vi "2) Programa Control.vi"(0 "VISA resource name":refnum<visa-resource-name>, 1 "error in (no error)":errorcluster) -> (3 "error out":errorcluster)   [LabVIEW 2019]
panel:
  out "Grafica arreglo":string[](array[string])
  in  "Tab Control":enum32{"Page 1"}(tab)
  in  "Refrescar":bool
  out "Gráfica":waveform(dbl)[](graph)
  in  "Guardar imagen":bool
  out "Voltaje":dbl[](array[numeric]) format="%#_4g"
  out "X":dbl[](array[numeric]) format="%#_4g"
  out "Cursores":string[](array[string])
  in  "Título":string
  in  "Guardar txt":bool
  in  "Guardar xls":bool
  in  "Detener":bool
  out "Multiplicadores":dbl[](array[numeric])
  out "Multiplicador":dbl
  out "Multiplicador2":ext
  in  "Acomplamiento":u16(ring) items=["AC", "DC", "GROUND"]
  in  "Atenuación":u16(ring) items=["x1", "x10", "x20", "x50", "x100", "x500", "x1000"]
  in  "Ancho de banda":u16(ring)=1 items=["ON", "OFF"]
  out "Comando 3":string
  in  "Posición vertical":i32(knob) scale=-5.0..5.0
  in  "Escala vertical (V)":u16(ring)=9 items=["2 mV", "5 mV", "10 mV", "20 mV", "50  mV", "100 mV", "200 mV", "500 mV", "1 V", "2 V", "5 V"]
  in  "Invertir canal 2":bool
  in  "Mayor Precisión":bool
  in  "Punto inicial de la onda":i32 min=0 max=2500 step=1
  in  "Punto final de la onda":i32=2500 min=0 max=2500 step=1
  in  "Nivel":ext
  in  "Mode":u16(ring) items=["Auto", "Normal"]
  in  "Estado":bool
  in  "Forzar":bool
  in  "Frecuencia":bool
  out "Comando final Trigger":string
  out "Tipo de trigger":string
  in  "Tipo de Trigger":enum32{"Flanco", "Video", "Pulso"}(tab)
  in  "Canal":u16(ring) items=["Canal 1", "Canal 2"]
  in  "Pendiente":u16(ring)=1 items=["Fall", "Rise"]
  in  "Acoplamiento":u16(ring) items=["AC", "DC", "Sin altas frecuencias DC", "Sin bajas frecuencias AC", "Baja sensibilidad DC"]
  in  "Sync":u16(ring) items=["Field", "Line", "Odd", "Even", "LineNum"]
  in  "Polaridad":u16(ring) items=["Inverted", "Normal"]
  in  "Líneas":dbl(knob) scale=0.0..525.0
  in  "Standard":u16(ring) items=["NTSC", "PAL"]
  in  "Canal":u16(ring) items=["Canal 1", "Canal 2"]
  in  "Width":dbl(knob) scale=3.3e-08..10.0
  in  "When":u16(ring) items=["Equal", "NotEqual", "Inside", "Outside"]
  in  "Polaritdad":u16(ring) items=["Positivo", "Negativo"]
  in  "Ancho":u16(ring) items=["Polarity", "When", "Width"]
  in  "Canal":u16(ring) items=["Canal 1", "Canal 2"]
  in  "Canal MATH":bool
  in  "Canal 1":bool
  in  "Canal 2":bool
  out "Comando 4":string
  out "Comando 2":string
  out "Comando 1":string
  in  "Invertir canal":bool
  in  "Posición horizontal":i32(knob) scale=-5.0..5.0
  in  "Posición vertical":i32(knob) scale=-5.0..5.0
  in  "Escala vertical (V)":u16(ring)=9 items=["2 mV", "5 mV", "10 mV", "20 mV", "50  mV", "100 mV", "200 mV", "500 mV", "1 V", "2 V", "5 V"]
  in  "Escala horizontal (s)":u16(ring)=14 items=["25 n", "50 n", "100 n", "250 n", "500 n", "1 u", "2,5 u", "5 u", "10 u", "25 u", "50 u", "100 u", "250 u", "500 u", "1 m", "2,5 m", "5 m", "10 m", "25 m", "50 m", "100 m", "250 m", "500 m", "1 ", "2,5", "5", "10", "25", "50"]
  in  "Operaciones con las \nseñales (Canal MATH)":u16(ring)=1 items=["CH1 + CH2"=1, "CH1 - CH2"=2, "CH2 - CH1"=3, "CH1 * CH2"=4]
  in  "Acomplamiento":u16(ring) items=["AC", "DC", "GROUND"]
  in  "Atenuación":u16(ring) items=["x1", "x10", "x20", "x50", "x100", "x500", "x1000"]
  in  "Ancho de banda":u16(ring)=1 items=["ON", "OFF"]
  out "Comando concatenado":string
  out "Comando final":string
  # "Opciones avanzadas (trigger)"
  # "Canal 1"
  # "Canal 2"
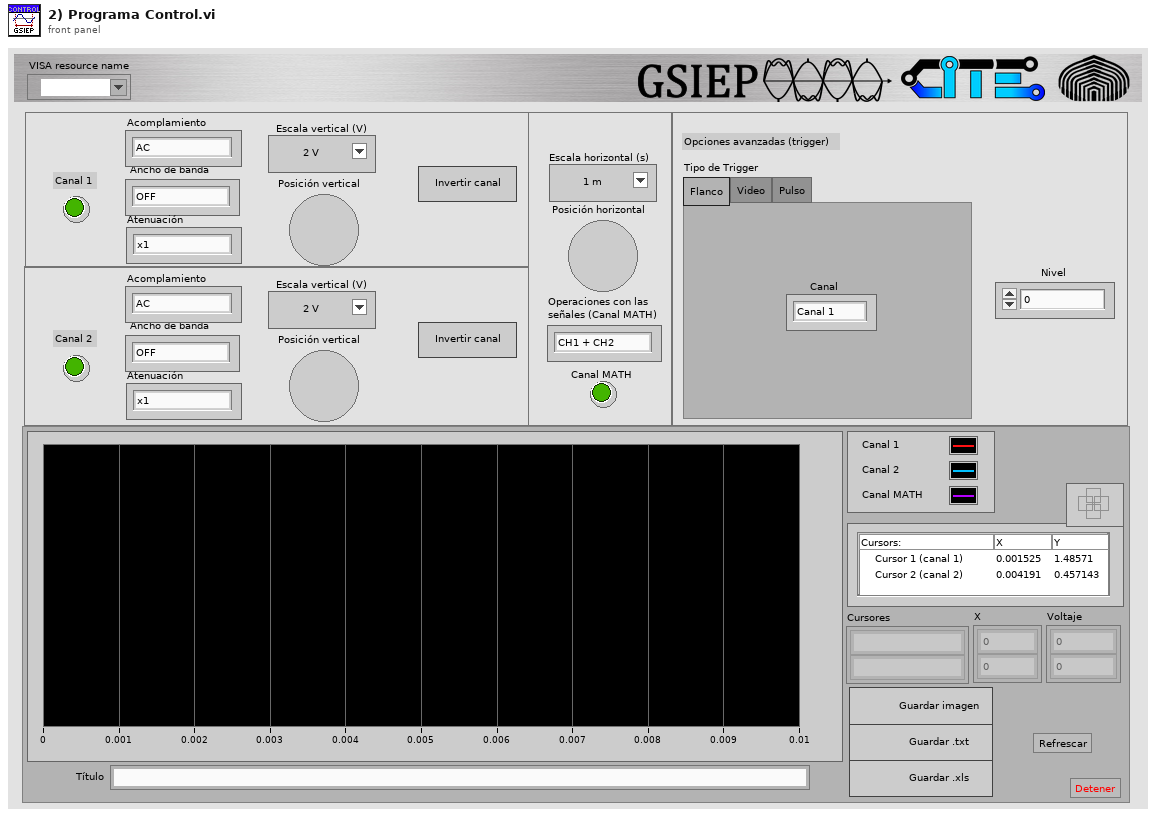
[diagram p1: front panel]
types:
  T1 = cluster{"Canal 1":bool, "Canal 2":bool, "Canal MATH":bool}
  T2 = typedef "LVCursorListTypeDef.ctl" = cluster{"Name":string, "Color":u32, "Style":u8, "Point Style":u8, "Name Visible":bool, "Allow Drag":bool, "Cursor Mode":u32, "Plot":i32, "Index":i32, "Position":cluster{"X":dbl, "Y":dbl}, "X Scale":u32, "Y Scale":u32, "Watch Plots":i32[], "Watch All Plots":bool, "Plot Area":i32, "Label Offset":cluster{"X":dbl, "Y":dbl}}[]
  T3 = typedef "imagedata.ctl" = cluster{"image type":i32, "image depth":i32, "image":u8[], "mask":u8[], "colors":u32[], "Rectangle":cluster{"left":i16, "top":i16, "right":i16, "bottom":i16}}
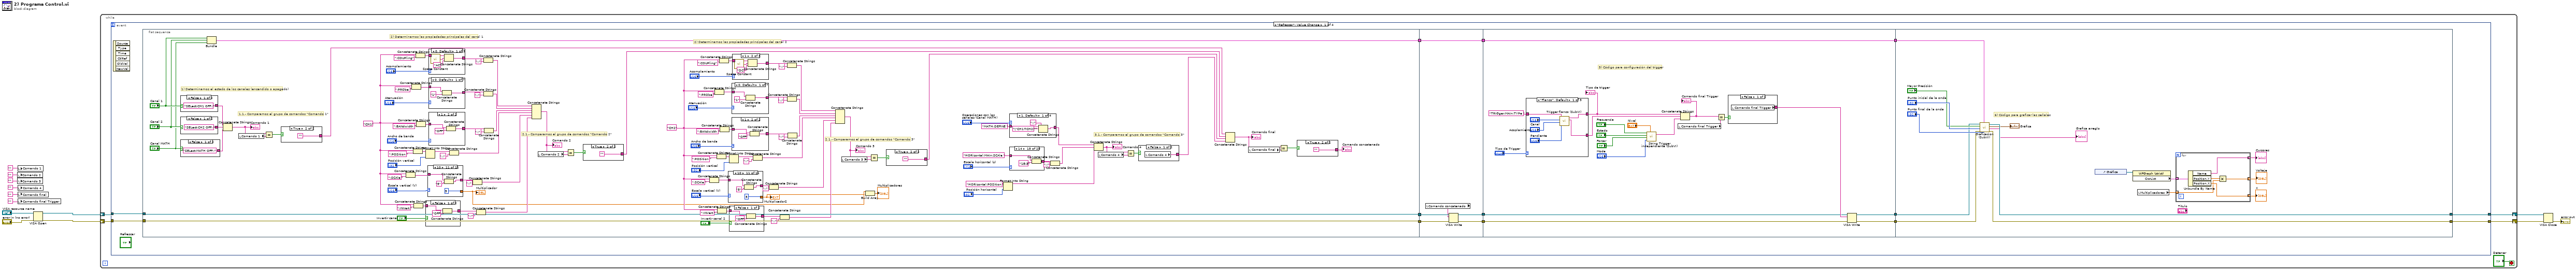
[diagram p0: block diagram]
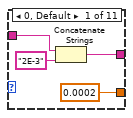
[diagram p2: hidden frame]
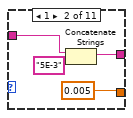
[diagram p3: hidden frame]
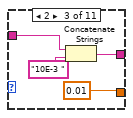
[diagram p4: hidden frame]
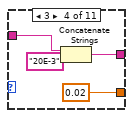
[diagram p5: hidden frame]
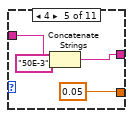
[diagram p6: hidden frame]
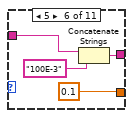
[diagram p7: hidden frame]
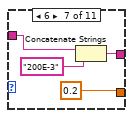
[diagram p8: hidden frame]
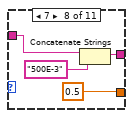
[diagram p9: hidden frame]
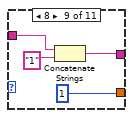
[diagram p10: hidden frame]
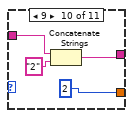
[diagram p11: hidden frame]
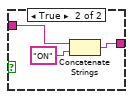
[diagram p12: hidden frame]
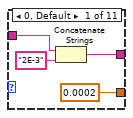
[diagram p13: hidden frame]
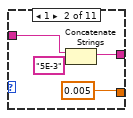
[diagram p14: hidden frame]
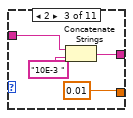
[diagram p15: hidden frame]
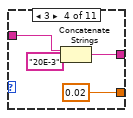
[diagram p16: hidden frame]
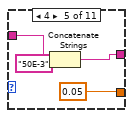
[diagram p17: hidden frame]
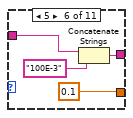
[diagram p18: hidden frame]
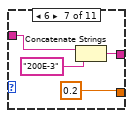
[diagram p19: hidden frame]
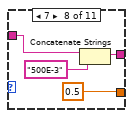
[diagram p20: hidden frame]
diagram:
  n1 = local write "Comando 2"("") -> ()
  n2 = local write "Comando 3"("") -> ()
  n3 = local write "Comando 1"("") -> ()
  n4 = local write "Comando 4"("") -> ()
  n5 = local write "Comando final"("") -> ()
  n6 = local write "Comando final Trigger"("") -> ()
  n7 = VISA Open(error in (no error)="error in (no error)", VISA resource name="VISA resource name") -> (VISA resource name=w2:refnum<visa-resource-name>, error out=w1:errorcluster)  [unwired: 3 in]
  n8 = while {
    shift-right: [w18] -> w13
    shift-left: w2 -> [w16]
    shift-right: [w17] -> w12
    shift-left: w1 -> [w15]
    stop <- "Detener" stop-if-true
    n9 = event shown="[0] \"Refrescar\": Value Change" {
      selector: _ -> [_ _ _ _]
      dyn-events: _ -> [_ _ _ _]
      timeout: _ -> [_ _ _ _]
      tunnel: w16 -> [w22 _ _ _]
      tunnel: w15 -> [w21 _ _ _]
      tunnel: [w20 _ _ _] -> w18
      tunnel: [w19 _ _ _] -> w17
      event "Refrescar": Value Change {
        n10 = event-data() -> ()  [unwired: 1 in, 6 out]
        n11 = flat-sequence {
          tunnel: [w147] -> w30
          tunnel: [w146] -> w29
          tunnel: [w85] -> w31
          tunnel: w22 -> [w147]
          tunnel: w21 -> [w146]
          tunnel: [w448] -> w28
          tunnel: [w447] -> w27
          tunnel: [w446] -> w26
          tunnel: w31 -> [w446]
          tunnel: w30 -> [w445]
          tunnel: w29 -> [w444]
          tunnel: w28 -> [w450]
          tunnel: w27 -> [w449]
          tunnel: w26 -> [w467]
          tunnel: [w453] -> w25
          tunnel: [w452] -> w24
          tunnel: [w467] -> w23
          tunnel: [w501] -> w19
          tunnel: [w502] -> w20
          tunnel: w25 -> [w504]
          tunnel: w24 -> [w503]
          tunnel: w23 -> [w500]
          frame #0 {
            w77 = "CH2"
            w81 = "CH1"
            # "2.1.- Comparamos el grupo de comandos \"Comando 3\""
            # "2) Determinamos las propiedades principales del canal 2"
            # "1) Determinamos el estado de los canales (encendido o apagado)"
            # "3.1.- Comparamos el grupo de comandos \"Comando 3\""
            # "2.1.- Comparamos el grupo de comandos \"Comando 2\""
            # "1.1.- Comparamos el grupo de comandos \"Comando 1\""
            # "2) Determinamos las propiedades principales del canal 1"
            n12 = case shown="False" "Canal 1" {
              tunnel: ["SELect:CH1 OFF;:" "SELect:CH1 ON;:"] -> w143
              frame False {
              }
              frame True {
              }
            }
            n13 = case shown="False" "Canal 2" {
              tunnel: ["SELect:CH2 OFF;:" "SELect:CH2 ON;:"] -> w142
              frame False {
              }
              frame True {
              }
            }
            n14 = case shown="False" "Canal MATH" {
              tunnel: ["SELect:MATH OFF;:" "SELect:MATH ON"] -> w141
              frame False {
              }
              frame True {
              }
            }
            n15 = Bundle("Canal 1"="Canal 1", "Canal 2"="Canal 2", "Canal MATH"="Canal MATH") -> (w85:T1)  [unwired: 1 in]
            n16 = Concatenate Strings(w143, w142, w141) -> (w140:string)
            "Comando 1" <- w140
            n17 = local read "Comando 1"() -> (w139:string)
            n18 = Equal?(x=w140, y=w139) -> (x = y?=w138:bool)
            n19 = case shown="True" w138 {
              tunnel: [w433 ""] -> w94
              frame False {
                n20 = local read "Comando 1"() -> (w433:string)
              }
              frame True {
              }
            }
            n21 = Concatenate Strings(w81, ":SCAle ") -> (w37:string)
            n22 = Concatenate Strings(w81, ":PRObe ") -> (w134:string)
            n23 = Concatenate Strings(w81, ":POSition ") -> (w107:string)
            n24 = Concatenate Strings(w81, ":INVert ") -> (w98:string)
            n25 = Concatenate Strings(w81, ":COUPling") -> (w137:string)
            n26 = Concatenate Strings(w81, ":BANdwidth ") -> (w132:string)
            n27 = Format Into String(initial string=w107, "Posición vertical") -> (resulting string=w112:string)  [unwired: 2 in, 1 out]
            n28 = case shown="False" "Invertir canal" {
              tunnel: w98 -> [w285 w288]
              tunnel: [w284 w287] -> w95
              frame False {
                n29 = Concatenate Strings(w285, "OFF") -> (w284:string)
              }
              frame True {
                n30 = Concatenate Strings(w288, "ON") -> (w287:string)
              }
            }
            n31 = case shown="10" "Escala vertical (V)" {
              tunnel: w37 -> [w151 w156 w159 w163 w167 w171 w174 w179 w183 w187 w191]
              tunnel: [w150 w154 w158 w162 w166 w170 w175 w178 w182 w186 w190] -> w35
              tunnel: [0.0002 0.005 0.01 0.02 0.05 0.1 0.2 0.5 1 2 5] -> w34
              frame 0, Default {
                n32 = Concatenate Strings(w151, "2E-3") -> (w150:string)
              }
              frame 1 {
                n33 = Concatenate Strings(w156, "5E-3") -> (w154:string)
              }
              frame 2 {
                n34 = Concatenate Strings(w159, "10E-3 ") -> (w158:string)
              }
              frame 3 {
                n35 = Concatenate Strings(w163, "20E-3") -> (w162:string)
              }
              frame 4 {
                n36 = Concatenate Strings(w167, "50E-3") -> (w166:string)
              }
              frame 5 {
                n37 = Concatenate Strings(w171, "100E-3") -> (w170:string)
              }
              frame 6 {
                n38 = Concatenate Strings(w174, "200E-3") -> (w175:string)
              }
              frame 7 {
                n39 = Concatenate Strings(w179, "500E-3") -> (w178:string)
              }
              frame 8 {
                n40 = Concatenate Strings(w183, "1") -> (w182:string)
              }
              frame 9 {
                n41 = Concatenate Strings(w187, "2") -> (w186:string)
              }
              frame 10 {
                n42 = Concatenate Strings(w191, "5") -> (w190:string)
              }
            }
            "Multiplicador" <- w34
            n43 = case shown="0, Default" "Atenuación" {
              tunnel: w134 -> [w401 w405 w407 w410 w413 w416 w419]
              tunnel: [w400 w403 w406 w409 w412 w415 w418] -> w123
              frame 0, Default {
                n44 = Concatenate Strings(w401, "1") -> (w400:string)
              }
              frame 1 {
                n45 = Concatenate Strings(w405, "10") -> (w403:string)
              }
              frame 2 {
                n46 = Concatenate Strings(w407, "20") -> (w406:string)
              }
              frame 3 {
                n47 = Concatenate Strings(w410, "50") -> (w409:string)
              }
              frame 4 {
                n48 = Concatenate Strings(w413, "100") -> (w412:string)
              }
              frame 5 {
                n49 = Concatenate Strings(w416, "500") -> (w415:string)
              }
              frame 6 {
                n50 = Concatenate Strings(w419, "1000") -> (w418:string)
              }
            }
            n51 = case shown="1" "Ancho de banda" {
              tunnel: w132 -> [w396 w399]
              tunnel: [w394 w397] -> w121
              frame 0, Default {
                n52 = Concatenate Strings(w396, "ON") -> (w394:string)
              }
              frame 1 {
                n53 = Concatenate Strings(w399, "OFF") -> (w397:string)
              }
            }
            n54 = case shown="0, Default" "Acomplamiento" {
              tunnel: w137 -> [w422 w425 w430]
              tunnel: [w421 w426 w429] -> w126
              frame 0, Default {
                n55 = call <vilib>:"Space Constant.vi"() -> ("String"=w423:string)
                n56 = Concatenate Strings(w422, w423, "AC") -> (w421:string)
              }
              frame 1 {
                n57 = call <vilib>:"Space Constant.vi"() -> ("String"=w427:string)
                n58 = Concatenate Strings(w425, w427, "DC") -> (w426:string)
              }
              frame 2 {
                n59 = call <vilib>:"Space Constant.vi"() -> ("String"=w431:string)
                n60 = Concatenate Strings(w430, w431, "GND") -> (w429:string)
              }
            }
            n61 = Concatenate Strings(w112, ";:") -> (w84:string)
            n62 = Concatenate Strings(w35, ";:") -> (w83:string)
            n63 = Concatenate Strings(w95, ";:") -> (w80:string)
            n64 = Concatenate Strings(w126, ";:") -> (w91:string)
            n65 = Concatenate Strings(w123, ";:") -> (w90:string)
            n66 = Concatenate Strings(w121, ";:") -> (w89:string)
            n67 = Concatenate Strings(w91, w90, w89, w84, w83, w80) -> (w118:string)
            "Comando 2" <- w118
            n68 = local read "Comando 2"() -> (w119:string)
            n69 = Equal?(x=w118, y=w119) -> (x = y?=w120:bool)
            n70 = case shown="True" w120 {
              tunnel: [w379 ""] -> w93
              frame False {
                n71 = local read "Comando 2"() -> (w379:string)
              }
              frame True {
              }
            }
            n72 = Concatenate Strings(w77, ":SCAle ") -> (w61:string)
            n73 = Concatenate Strings(w77, ":PRObe ") -> (w42:string)
            n74 = Concatenate Strings(w77, ":POSition ") -> (w64:string)
            n75 = Concatenate Strings(w77, ":INVert ") -> (w68:string)
            n76 = Concatenate Strings(w77, ":COUPling") -> (w39:string)
            n77 = Concatenate Strings(w77, ":BANdwidth ") -> (w44:string)
            n78 = case shown="10" "Escala vertical (V)" {
              tunnel: w61 -> [w201 w206 w209 w213 w217 w221 w224 w229 w233 w237 w241]
              tunnel: [w200 w204 w208 w212 w216 w220 w225 w228 w232 w236 w240] -> w65
              tunnel: [0.0002 0.005 0.01 0.02 0.05 0.1 0.2 0.5 1 2 5] -> w33
              frame 0, Default {
                n79 = Concatenate Strings(w201, "2E-3") -> (w200:string)
              }
              frame 1 {
                n80 = Concatenate Strings(w206, "5E-3") -> (w204:string)
              }
              frame 2 {
                n81 = Concatenate Strings(w209, "10E-3 ") -> (w208:string)
              }
              frame 3 {
                n82 = Concatenate Strings(w213, "20E-3") -> (w212:string)
              }
              frame 4 {
                n83 = Concatenate Strings(w217, "50E-3") -> (w216:string)
              }
              frame 5 {
                n84 = Concatenate Strings(w221, "100E-3") -> (w220:string)
              }
              frame 6 {
                n85 = Concatenate Strings(w224, "200E-3") -> (w225:string)
              }
              frame 7 {
                n86 = Concatenate Strings(w229, "500E-3") -> (w228:string)
              }
              frame 8 {
                n87 = Concatenate Strings(w233, "1") -> (w232:string)
              }
              frame 9 {
                n88 = Concatenate Strings(w237, "2") -> (w236:string)
              }
              frame 10 {
                n89 = Concatenate Strings(w241, "5") -> (w240:string)
              }
            }
            "Multiplicador2" <- w33
            n90 = Format Into String(initial string=w64, "Posición vertical") -> (resulting string=w59:string)  [unwired: 2 in, 1 out]
            n91 = case shown="False" "Invertir canal 2" {
              tunnel: w68 -> [w194 w197]
              tunnel: [w193 w196] -> w71
              frame False {
                n92 = Concatenate Strings(w194, "OFF") -> (w193:string)
              }
              frame True {
                n93 = Concatenate Strings(w197, "ON") -> (w196:string)
              }
            }
            n94 = case shown="0, Default" "Atenuación" {
              tunnel: w42 -> [w252 w256 w258 w261 w264 w267 w270]
              tunnel: [w251 w254 w257 w260 w263 w266 w269] -> w51
              frame 0, Default {
                n95 = Concatenate Strings(w252, "1") -> (w251:string)
              }
              frame 1 {
                n96 = Concatenate Strings(w256, "10") -> (w254:string)
              }
              frame 2 {
                n97 = Concatenate Strings(w258, "20") -> (w257:string)
              }
              frame 3 {
                n98 = Concatenate Strings(w261, "50") -> (w260:string)
              }
              frame 4 {
                n99 = Concatenate Strings(w264, "100") -> (w263:string)
              }
              frame 5 {
                n100 = Concatenate Strings(w267, "500") -> (w266:string)
              }
              frame 6 {
                n101 = Concatenate Strings(w270, "1000") -> (w269:string)
              }
            }
            n102 = case shown="1" "Ancho de banda" {
              tunnel: w44 -> [w247 w250]
              tunnel: [w245 w248] -> w53
              frame 0, Default {
                n103 = Concatenate Strings(w247, "ON") -> (w245:string)
              }
              frame 1 {
                n104 = Concatenate Strings(w250, "OFF") -> (w248:string)
              }
            }
            n105 = case shown="1" "Acomplamiento" {
              tunnel: w39 -> [w273 w276 w281]
              tunnel: [w272 w277 w280] -> w48
              frame 0, Default {
                n106 = call <vilib>:"Space Constant.vi"() -> ("String"=w274:string)
                n107 = Concatenate Strings(w273, w274, "AC") -> (w272:string)
              }
              frame 1 {
                n108 = call <vilib>:"Space Constant.vi"() -> ("String"=w278:string)
                n109 = Concatenate Strings(w276, w278, "DC") -> (w277:string)
              }
              frame 2 {
                n110 = call <vilib>:"Space Constant.vi"() -> ("String"=w282:string)
                n111 = Concatenate Strings(w281, w282, "GND") -> (w280:string)
              }
            }
            n112 = Concatenate Strings(w59, ";:") -> (w75:string)
            n113 = Concatenate Strings(w65, ";:") -> (w76:string)
            n114 = Concatenate Strings(w71, ";:") -> (w78:string)
            n115 = Concatenate Strings(w48, ";:") -> (w72:string)
            n116 = Concatenate Strings(w51, ";:") -> (w73:string)
            n117 = Concatenate Strings(w53, ";:") -> (w74:string)
            n118 = Concatenate Strings(w72, w73, w74, w75, w76, w78) -> (w56:string)
            "Comando 3" <- w56
            n119 = local read "Comando 3"() -> (w55:string)
            n120 = Build Array(w34, w33) -> (→"Multiplicadores":dbl[])
            n121 = Equal?(x=w56, y=w55) -> (x = y?=w54:bool)
            n122 = case shown="True" w54 {
              tunnel: [w243 ""] -> w38
              frame False {
                n123 = local read "Comando 3"() -> (w243:string)
              }
              frame True {
              }
            }
            n124 = Format Into String(initial string="HORizontal:POSition ", "Posición horizontal") -> (resulting string=w114:string)  [unwired: 2 in, 1 out]
            n125 = case shown="1, Default" "Operaciones con las \nseñales (Canal MATH)" {
              tunnel: "MATH:DEFINE " -> [w384 w387 w389 w392]
              tunnel: [w382 w386 w388 w391] -> w82
              frame 1, Default {
                n126 = Concatenate Strings(w384, "\"CH1+CH2\"", ";:" ("string")) -> (w382:string)
              }
              frame 2 {
                n127 = Concatenate Strings(w387, "\"CH1-CH2\"") -> (w386:string)
              }
              frame 3 {
                n128 = Concatenate Strings(w389, "\"CH2-CH1\"") -> (w388:string)
              }
              frame 4 {
                n129 = Concatenate Strings(w392, "\"CH1*CH2\"") -> (w391:string)
              }
            }
            n130 = case shown="14" "Escala horizontal (s)" {
              tunnel: "HORizontal:MAIn:SCAle " -> [w293 w297 w299 w302 w305 w308 w311 w314 w317 w320 w323 w325 w328 w331 w334 w337 w340 w343 w346 w349 w352 w355 w358 w361 w364 w367 w370 w373 w376]
              tunnel: [w292 w295 w298 w301 w304 w307 w312 w313 w316 w319 w322 w326 w329 w332 w335 w338 w341 w344 w347 w350 w353 w356 w359 w362 w365 w368 w371 w374 w377] -> w105
              frame 0, Default {
                n131 = Concatenate Strings(w293, "25E-9") -> (w292:string)
              }
              frame 1 {
                n132 = Concatenate Strings(w297, "50E-9") -> (w295:string)
              }
              frame 2 {
                n133 = Concatenate Strings(w299, "100E-9") -> (w298:string)
              }
              frame 3 {
                n134 = Concatenate Strings(w302, "250E-9") -> (w301:string)
              }
              frame 4 {
                n135 = Concatenate Strings(w305, "500E-9") -> (w304:string)
              }
              frame 5 {
                n136 = Concatenate Strings(w308, "1E-6") -> (w307:string)
              }
              frame 6 {
                n137 = Concatenate Strings(w311, "2.5E-6") -> (w312:string)
              }
              frame 7 {
                n138 = Concatenate Strings(w314, "5E-6") -> (w313:string)
              }
              frame 8 {
                n139 = Concatenate Strings(w317, "10E-6") -> (w316:string)
              }
              frame 9 {
                n140 = Concatenate Strings(w320, "25E-6") -> (w319:string)
              }
              frame 10 {
                n141 = Concatenate Strings(w323, "50E-6") -> (w322:string)
              }
              frame 11 {
                n142 = Concatenate Strings(w325, "100E-6") -> (w326:string)
              }
              frame 12 {
                n143 = Concatenate Strings(w328, "250E-6") -> (w329:string)
              }
              frame 13 {
                n144 = Concatenate Strings(w331, "500E-6") -> (w332:string)
              }
              frame 14 {
                n145 = Concatenate Strings(w334, "1E-3") -> (w335:string)
              }
              frame 15 {
                n146 = Concatenate Strings(w337, "2.5E-3") -> (w338:string)
              }
              frame 16 {
                n147 = Concatenate Strings(w340, "5E-3") -> (w341:string)
              }
              frame 17 {
                n148 = Concatenate Strings(w343, "10E-3") -> (w344:string)
              }
              frame 18 {
                n149 = Concatenate Strings(w346, "25E-3") -> (w347:string)
              }
              frame 19 {
                n150 = Concatenate Strings(w349, "50E-3") -> (w350:string)
              }
              frame 20 {
                n151 = Concatenate Strings(w352, "100E-3") -> (w353:string)
              }
              frame 21 {
                n152 = Concatenate Strings(w355, "250E-3") -> (w356:string)
              }
              frame 22 {
                n153 = Concatenate Strings(w358, "500E-3") -> (w359:string)
              }
              frame 23 {
                n154 = Concatenate Strings(w361, "1E0") -> (w362:string)
              }
              frame 24 {
                n155 = Concatenate Strings(w364, "2.5E0") -> (w365:string)
              }
              frame 25 {
                n156 = Concatenate Strings(w367, "5E0") -> (w368:string)
              }
              frame 26 {
                n157 = Concatenate Strings(w370, "10E0") -> (w371:string)
              }
              frame 27 {
                n158 = Concatenate Strings(w373, "25E0") -> (w374:string)
              }
              frame 28 {
                n159 = Concatenate Strings(w376, "50E0") -> (w377:string)
              }
            }
            n160 = Concatenate Strings(w105, ";:") -> (w104:string)
            n161 = Concatenate Strings(w82, w104, w114) -> (w100:string)
            "Comando 4" <- w100
            n162 = local read "Comando 4"() -> (w102:string)
            n163 = Equal?(x=w100, y=w102) -> (x = y?=w101:bool)
            n164 = case shown="False" w101 {
              tunnel: [w290 ""] -> w79
              frame False {
                n165 = local read "Comando 4"() -> (w290:string)
              }
              frame True {
              }
            }
            n166 = Concatenate Strings(w94, w93, w38, w79) -> (w92:string)
            "Comando final" <- w92
            n167 = local read "Comando final"() -> (w145:string)
            n168 = Equal?(x=w92, y=w145) -> (x = y?=w148:bool)
            n169 = case shown="True" w148 {
              tunnel: [w441 ""] -> w144
              frame False {
                n170 = local read "Comando final"() -> (w441:string)
              }
              frame True {
              }
            }
            "Comando concatenado" <- w144
          }
          frame #1 {
            n171 = local read "Comando concatenado"() -> (w443:string)
            n172 = VISA Write(VISA resource name=w445, write buffer=w443, error in (no error)=w444) -> (VISA resource name out=w448:refnum<visa-resource-name>, error out=w447:errorcluster)  [unwired: 1 out]
          }
          frame #2 {
            # "5) Código para configuración del trigger"
            n173 = case shown="\"Flanco\", Default" "Tipo de Trigger" {
              tunnel: "TRIGger:MAIn:TYPe " -> [w474 w480 w491]
              tunnel: [w475 w482 w490] -> w455
              tunnel: [w470 w481 w489] -> w456
              frame "Flanco", Default {
                n174 = call "Trigger flanco (SubVI).vi"("Slope"="Pendiente", "Acoplamiento"="Acoplamiento", "Canal"="Canal", "String de Entrada"=w474) -> ("String de Salida"=w470:string, "String de tipo"=w475:string)  [unwired: 6 in]
              }
              frame "Video" {
                n175 = call "Trigger Video (SubVI).vi"("Sync"="Sync", "Lines"="Líneas", "Standard"="Standard", "Polarity"="Polaridad", "Canal"="Canal", "String de Entrada"=w480) -> ("String de Salida"=w481:string, "String de Tipo"=w482:string)  [unwired: 4 in]
              }
              frame "Pulso" {
                n176 = call "Trigger Pulso (SubVI).vi"("Polarity"="Polaritdad", "Width"="Width", "When"="When", "Ancho"="Ancho", "Canal"="Canal", "String de Entrada"=w491) -> ("String de Salida"=w489:string, "String de Tipo"=w490:string)  [unwired: 4 in]
              }
            }
            "Tipo de trigger" <- w455
            n177 = call "String Trigger independiente (SubVI).vi"("Nivel"="Nivel", "Mode"="Mode", "Force"="Forzar", "State"="Estado", "Frecuency"="Frecuencia") -> ("String trigges independiente"=w466:string)  [unwired: 2 in]
            n178 = local read "Comando final Trigger"() -> (w457:string)
            n179 = Concatenate Strings(w455, w456, w466) -> (w454:string)
            "Comando final Trigger" <- w454
            n180 = Equal?(x=w454, y=w457) -> (x = y?=w458:bool)
            n181 = case shown="False" w458 {
              tunnel: [w468 ""] -> w451
              frame False {
                n182 = local read "Comando final Trigger"() -> (w468:string)
              }
              frame True {
              }
            }
            n183 = VISA Write(VISA resource name=w450, write buffer=w451, error in (no error)=w449) -> (VISA resource name out=w453:refnum<visa-resource-name>, error out=w452:errorcluster)  [unwired: 1 out]
          }
          frame #3 {
            # "6) Código para graficar las señales"
            n184 = call "Graficacion (SubVI).vi"("Punto final de la onda"="Punto final de la onda", "Estados de los canales"=w500, "error in (no error)"=w503, "Punto inicial de la onda"="Punto inicial de la onda", "Mayor Precisión"="Mayor Precisión", "VISA Refnum in"=w504) -> ("error out"=w501:errorcluster, "Array"=→"Grafica arreglo":string[], "Gráfica"=→"Gráfica":waveform(dbl)[], "VISA Refnum out"=w502:refnum<visa-resource-name>)  [unwired: 2 in]
            n185 = control-ref of="Gráfica"() -> (w492:refnum<vi>)
            n186 = property class="WFGraph (strict)"(reference=w492) -> ("CrsrList"=w498:T2)  [unwired: 1 in, 2 out]
            n187 = local read "Multiplicadores"() -> (w495:dbl[])
            n188 = for {
              tunnel: w498 -> [w513] mode=indexing
              tunnel: [w512] -> w496 mode=indexing
              tunnel: [w511] -> w497 mode=indexing
              tunnel: w495 -> [w509] mode=indexing
              tunnel: [w508] -> w494 mode=indexing
              n189 = Unbundle By Name(w513) -> ("Name"=w512:string, "Position.Y"=w510:dbl, "Position.X"=w511:dbl)
              n190 = Multiply(x=w510, y=w509) -> (x*y=w508:dbl)
            }
            "Voltaje" <- w494
            "X" <- w497
            "Cursores" <- w496
          }
        }
      }
      event "Guardar txt": Value Change {
        n191 = event-data() -> ()  [unwired: 1 in, 6 out]
        n192 = local read "Grafica arreglo"() -> (w514:string[])
        n193 = case shown="False" "Guardar txt" {
          tunnel: w514 -> [_ w518]
          frame False {
          }
          frame True {
            n194 = File Dialog(6:"*.txt") -> (0:w517:errorcluster, 3:w519:path)  [unwired: 6 in, 2 out]
            n195 = Write to Text File(file (use dialog)=w519, text=w518, error in=w517) -> (refnum out=w520:refnum<file>, error out=w521:errorcluster)  [unwired: 1 in, 1 out]
            n196 = Close File(refnum=w520, error in=w521) -> ()  [unwired: 2 out]
          }
        }
      }
      event "Guardar xls": Value Change {
        n197 = event-data() -> ()  [unwired: 1 in, 6 out]
        n198 = local read "Grafica arreglo"() -> (w522:string[])
        n199 = case shown="False" "Guardar xls" {
          tunnel: w522 -> [_ w527]
          frame False {
          }
          frame True {
            n200 = File Dialog(6:"*.xls") -> (0:w525:errorcluster, 3:w526:path)  [unwired: 6 in, 2 out]
            n201 = Write to Text File(file (use dialog)=w526, text=w527, error in=w525) -> (refnum out=w529:refnum<file>, error out=w528:errorcluster)  [unwired: 1 in, 1 out]
            n202 = Close File(refnum=w529, error in=w528) -> ()  [unwired: 2 out]
          }
        }
      }
      event "Guardar imagen": Value Change {
        n203 = event-data() -> ()  [unwired: 1 in, 6 out]
        n204 = case shown="True" "Guardar imagen" {
          frame False {
          }
          frame True {
            n205 = File Dialog(6:"*.png" ("pattern")) -> (1:w532:bool, 3:w533:path)  [unwired: 6 in, 2 out]
            n206 = case shown="False" w532 {
              tunnel: w533 -> [w536 _]
              frame False {
                n207 = invoke on="Tab Control" class="TabCtl (strict)" method="Get Image"("image depth"=24) -> ("image data"=w535:T3)  [unwired: 5 in, 5 out]
                n208 = call <vilib>:"Write PNG File.vi"("image data"=w535, "path to PNG file"=w536) -> ()  [unwired: 8 in, 2 out]
              }
              frame True {
              }
            }
          }
        }
      }
    }
  }
  n209 = VISA Close(VISA resource name=w13, error in (no error)=w12) -> (error out=→"error out":errorcluster)
